vi "Create Client from TCP.vi"(8 "error in (no error)":errorcluster, 9 "URI":refnum<class "URI.lvclass">, 10 "TCP Connection":refnum<k5>, 11 "Websocket Server in":refnum<class "Websocket Server.lvclass">) -> (0 "error out":errorcluster, 3 "Websocket Server out":refnum<class "Websocket Server.lvclass">)   [LabVIEW 2020, in "Stream-Websocket.lvlib" / "Websocket Server.lvclass"]
uses:
  Websocket Server.lvclass
  <vilib>/IlluminatedG/lv-stream/URI/URI.lvclass
  Websocket Server.lvclass/Websocket Server.ctl
  Websocket Client/Websocket Client.lvclass
  C:/Program Files (x86)/National Instruments/LabVIEW 2020/vi.lib/IlluminatedG/lv-stream/Endpoint/Endpoint.lvclass
  C:/dev/illuminated-g/lv-stream-websocket/Stream-Websocket/Websocket Server/Websocket Server.lvclass
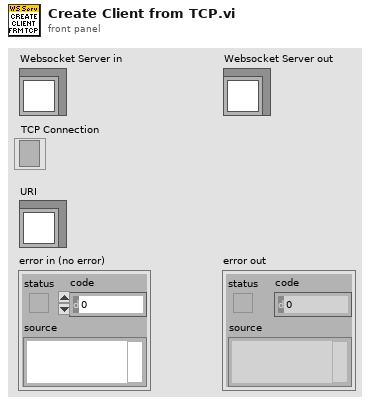
[diagram p1: front panel]
types:
  T1 = typedef "Stream-Websocket.lvlib/Listener Result.ctl" = cluster{"Status":T2, "Client":refnum<class "Websocket Client.lvclass">}
  T2 = typedef "Stream-Websocket.lvlib/Listener Status.ctl" = enum16{"Successful", "Unsuccessful"}
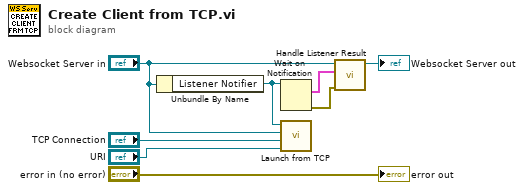
[diagram p0: block diagram]
diagram:
  n1 = Unbundle By Name("Websocket Server in") -> ("Listener Notifier"=w3:refnum<notifier>)
  n2 = Wait on Notification(notifier=w3) -> (notification=w5:T1, error out=w4:errorcluster)  [unwired: 3 in, 2 out]
  n3 = call "Launch from TCP.vi"("URI"="URI", "TCP Connection"="TCP Connection", "Server Endpoint"="Websocket Server in", "Listener Notifier"=w3) -> ()  [unwired: 7 in, 1 out]
  n4 = call "Handle Listener Result.vi"("error in (no error)"=w4, "Listener Result"=w5, "Websocket Server in"="Websocket Server in") -> ("Websocket Server out"=→"Websocket Server out":refnum<class "Websocket Server.lvclass">)  [unwired: 6 in, 2 out]
  "error out" <- "error in (no error)"
